vi "test_read-nmea-data2.vi"() -> ()   [LabVIEW 2019] (continued)
3,12,06,19,05,17,09,04,02,,,,,1.18,0.64,0.99,1*0A\n\t\n15:10:54.32\tF9P\t$GNGSA,A,3,85,71,84,,,,,,,,,,1.18,0.64,0.99,2*0F\n\t\n15:10:54.34\tF9P\t$GNGSA,A,3,36,19,11,04,09,12,,,,,,,1.18,0.64,0.99,3*0A\n\t\n15:10:54.37\tF9P\t$GNGSA,A,3,14,11,33,,,,,,,,,,1.18,0.64,0.99,4*0B\n\t\n15:10:54.39\tF9P\t$GPGSV,3,1,09,02,54,318,30,04,18,044,13,05,37,247,22,06,64,047,29,1*66\n\t\n15:10:54.41\tF9P\t$GPGSV,3,2,09,09,45,074,18,12,24,277,23,17,33,153,26,19,53,157,24,1*66\n\t\n15:10:54.43\tF9P\t$GPGSV,3,3,09,25,12,307,17,1*5B\n\t\n15:10:54.45\tF9P\t$GPGSV,3,1,09,02,54,318,,04,18,044,,05,37,247,,06,64,047,17,6*6D\n\t\n15:10:54.47\tF9P\t$GPGSV,3,2,09,09,45,074,,12,24,277,,17,33,153,15,19,53,157,,6*6F\n\t\n15:10:54.49\tF9P\t$GPGSV,3,3,09,25,12,307,,6*5A\n\t\n15:10:54.51\tF9P\t$GLGSV,2,1,08,69,12,031,,70,72,041,,71,51,205,16,72,03,209,,1*75\n\t\n15:10:54.53\tF9P\t$GLGSV,2,2,08,77,01,326,,84,20,122,11,85,70,065,23,86,36,330,,1*7A\n\t\n15:10:54.55\tF9P\t$GLGSV,2,1,08,69,12,031,,70,72,041,,71,51,205,23,72,03,209,,3*71\n\t\n15:10:54.57\tF9P\t$GLGSV,2,2,08,77,01,326,,84,20,122,15,85,70,065,21,86,36,330,,3*7E\n\t\n15:10:54.59\tF9P\t$GAGSV,2,1,08,02,09,298,11,04,66,119,25,09,31,193,21,11,71,357,20,7*7C\n\t\n15:10:54.61\tF9P\t$GAGSV,2,2,08,12,40,102,20,19,27,045,14,25,09,249,,36,25,308,10,7*7D\n\t\n15:10:54.63\tF9P\t$GAGSV,2,1,08,02,09,298,,04,66,119,24,09,31,193,,11,71,357,,2*79\n\t\n15:10:54.65\tF9P\t$GAGSV,2,2,08,12,40,102,29,19,27,045,,25,09,249,,36,25,308,,2*75\n\t\n15:10:54.67\tF9P\t$GBGSV,1,1,03,11,50,131,22,14,87,138,22,33,60,219,23,1*4E\n\t\n15:10:54.69\tF9P\t$GBGSV,1,1,03,11,50,131,35,14,87,138,15,33,60,219,,3*4F\n\t\n15:10:54.71\tF9P\t$GNGLL,3723.55311,N,12656.88974,E,061056.00,A,A*79\n\t\n15:10:54.73\tF9P\t\t\n15:10:54.75\tF9P\t\t\n15:10:54.77\tF9P\t\t\n15:10:54.79\tF9P\t\t\n15:10:54.81\tF9P\t\t\n15:10:54.83\tF9P\t\t\n15:10:54.85\tF9P\t\t\n15:10:54.87\tF9P\t\t\n15:10:54.89\tF9P\t\t\n15:10:54.91\tF9P\t\t\n15:10:54.93\tF9P\t\t\n15:10:54.95\tF9P\t\t\n15:10:54.97\tF9P\t\t\n15:10:54.99\tF9P\t\t\n15:10:55.01\tF9P\t\t\n15:10:55.03\tF9P\t\t\n15:10:55.05\tF9P\t\t\n15:10:55.07\tF9P\t\t\n15:10:55.09\tF9P\t\t\n15:10:55.11\tF9P\t\t\n15:10:55.13\tF9P\t\t\n15:10:55.15\tF9P\t\t\n15:10:55.17\tF9P\t\t\n15:10:55.19\tF9P\t\t\n15:10:55.21\tF9P\t\t\n15:10:55.23\tF9P\t\t\n15:10:55.25\tF9P\t$GNRMC,061057.00,A,3723.55267,N,12656.89064,E,2.717,135.11,250720,,,A,V*0A\n\t\n15:10:55.27\tF9P\t$GNVTG,135.11,T,,M,2.717,N,5.032,K,A*23\n\t\n15:10:55.29\tF9P\t$GNGGA,061057.00,3723.55267,N,12656.89064,E,1,12,0.64,66.5,M,18.5,M,,*7C\n\t\n15:10:55.31\tF9P\t$GNGSA,A,3,12,06,19,05,17,09,04,02,,,,,1.18,0.64,0.99,1*0A\n\t\n15:10:55.33\tF9P\t$GNGSA,A,3,85,71,84,,,,,,,,,,1.18,0.64,0.99,2*0F\n\t\n15:10:55.35\tF9P\t$GNGSA,A,3,36,19,11,04,09,12,,,,,,,1.18,0.64,0.99,3*0A\n\t\n15:10:55.37\tF9P\t$GNGSA,A,3,14,11,33,,,,,,,,,,1.18,0.64,0.99,4*0B\n\t\n15:10:55.39\tF9P\t$GPGSV,3,1,09,02,54,318,35,04,18,044,13,05,37,247,21,06,64,047,29,1*60\n\t\n15:10:55.41\tF9P\t$GPGSV,3,2,09,09,45,074,19,12,24,277,23,17,33,153,26,19,53,157,23,1*60\n\t\n15:10:55.43\tF9P\t$GPGSV,3,3,09,25,12,307,18,1*54\n\t\n15:10:55.45\tF9P\t$GPGSV,3,1,09,02,54,318,,04,18,044,,05,37,247,,06,64,047,17,6*6D\n\t\n15:10:55.47\tF9P\t$GPGSV,3,2,09,09,45,074,,12,24,277,,17,33,153,16,19,53,157,,6*6C\n\t\n15:10:55.49\tF9P\t$GPGSV,3,3,09,25,12,307,,6*5A\n\t\n15:10:55.51\tF9P\t$GLGSV,2,1,08,69,12,031,,70,72,041,,71,51,205,16,72,03,209,,1*75\n\t\n15:10:55.53\tF9P\t$GLGSV,2,2,08,77,01,326,,84,20,122,10,85,70,065,22,86,36,330,,1*7A\n\t\n15:10:55.55\tF9P\t$GLGSV,2,1,08,69,12,031,,70,72,041,,71,51,205,23,72,03,209,,3*71\n\t\n15:10:55.57\tF9P\t$GLGSV,2,2,08,77,01,326,,84,20,122,17,85,70,065,22,86,36,330,,3*7F\n\t\n15:10:55.59\tF9P\t$GAGSV,2,1,08,02,09,298,09,04,66,119,31,09,31,193,21,11,71,357,21,7*71\n\t\n15:10:55.61\tF9P\t$GAGSV,2,2,08,12,40,102,20,19,27,045,10,25,09,249,,36,25,308,10,7*79\n\t\n15:10:55.63\tF9P\t$GAGSV,2,1,08,02,09,298,,04,66,119,30,09,31,193,,11,71,357,,2*7C\n\t\n15:10:55.65\tF9P\t$GAGSV,2,2,08,12,40,102,26,19,27,045,,25,09,249,,36,25,308,,2*7A\n\t\n15:10:55.67\tF9P\t$GBGSV,1,1,03,11,50,131,24,14,87,138,21,33,60,219,23,1*4B\n\t\n15:10:55.69\tF9P\t$GBGSV,1,1,03,11,50,131,33,14,87,138,18,33,60,219,,3*44\n\t\n15:10:55.71\tF9P\t$GNGLL,3723.55267,N,12656.89064,E,061057.00,A,A*71\n\t\n15:10:55.73\tF9P\t\t\n15:10:55.75\tF9P\t\t\n15:10:55.77\tF9P\t\t\n15:10:55.79\tF9P\t\t\n15:10:55.81\tF9P\t\t\n15:10:55.83\tF9P\t\t\n15:10:55.85\tF9P\t\t\n15:10:55.87\tF9P\t\t\n15:10:55.89\tF9P\t\t\n15:10:55.91\tF9P\t\t\n15:10:55.93\tF9P\t\t\n15:10:55.95\tF9P\t\t\n15:10:55.97\tF9P\t\t\n15:10:55.99\tF9P\t\t\n15:10:56.01\tF9P\t\t\n15:10:56.03\tF9P\t\t\n15:10:56.05\tF9P\t\t\n15:10:56.07\tF9P\t\t\n15:10:56.09\tF9P\t\t\n15:10:56.11\tF9P\t\t\n15:10:56.13\tF9P\t\t\n15:10:56.15\tF9P\t\t\n15:10:56.17\tF9P\t\t\n15:10:56.19\tF9P\t\t\n15:10:56.21\tF9P\t\t\n15:10:56.23\tF9P\t\t\n15:10:56.25\tF9P\t$GNRMC,061058.00,A,3723.55188,N,12656.89111,E,3.072,148.78,250720,,,A,V*04\n\t\n15:10:56.27\tF9P\t$GNVTG,148.78,T,,M,3.072,N,5.690,K,A*2D\n\t\n15:10:56.29\tF9P\t$GNGGA,061058.00,3723.55188,N,12656.89111,E,1,12,0.76,66.2,M,18.5,M,,*76\n\t\n15:10:56.31\tF9P\t$GNGSA,A,3,12,06,19,05,17,09,04,02,,,,,1.40,0.76,1.18,1*0C\n\t\n15:10:56.33\tF9P\t$GNGSA,A,3,85,71,84,,,,,,,,,,1.40,0.76,1.18,2*09\n\t\n15:10:56.35\tF9P\t$GNGSA,A,3,36,19,11,04,09,12,,,,,,,1.40,0.76,1.18,3*0C\n\t\n15:10:56.37\tF9P\t$GNGSA,A,3,14,11,33,,,,,,,,,,1.40,0.76,1.18,4*0D\n\t\n15:10:56.39\tF9P\t$GPGSV,3,1,09,02,54,318,34,04,18,044,10,05,37,247,22,06,64,047,28,1*60\n\t\n15:10:56.41\tF9P\t$GPGSV,3,2,09,09,45,074,19,12,24,277,23,17,33,153,25,19,53,157,22,1*62\n\t\n15:10:56.43\tF9P\t$GPGSV,3,3,09,25,12,307,17,1*5B\n\t\n15:10:56.45\tF9P\t$GPGSV,3,1,09,02,54,318,,04,18,044,,05,37,247,,06,64,047,16,6*6C\n\t\n15:10:56.47\tF9P\t$GPGSV,3,2,09,09,45,074,,12,24,277,,17,33,153,18,19,53,157,,6*62\n\t\n15:10:56.49\tF9P\t$GPGSV,3,3,09,25,12,307,,6*5A\n\t\n15:10:56.51\tF9P\t$GLGSV,2,1,08,69,12,031,,70,72,041,,71,51,205,19,72,03,209,,1*7A\n\t\n15:10:56.53\tF9P\t$GLGSV,2,2,08,77,01,326,,84,20,122,09,85,70,065,22,86,36,330,,1*72\n\t\n15:10:56.55\tF9P\t$GLGSV,2,1,08,69,12,031,,70,72,041,,71,51,205,21,72,03,209,,3*73\n\t\n15:10:56.57\tF9P\t$GLGSV,2,2,08,77,01,326,,84,20,122,18,85,70,065,20,86,36,330,,3*72\n\t\n15:10:56.59\tF9P\t$GAGSV,2,1,08,02,09,298,11,04,66,119,25,09,31,193,20,11,71,357,22,7*7F\n\t\n15:10:56.61\tF9P\t$GAGSV,2,2,08,12,40,102,19,19,27,045,13,25,09,249,,36,25,308,14,7*74\n\t\n15:10:56.63\tF9P\t$GAGSV,2,1,08,02,09,298,,04,66,119,27,09,31,193,,11,71,357,,2*7A\n\t\n15:10:56.65\tF9P\t$GAGSV,2,2,08,12,40,102,26,19,27,045,,25,09,249,,36,25,308,,2*7A\n\t\n15:10:56.67\tF9P\t$GBGSV,1,1,03,11,50,131,24,14,87,138,21,33,60,219,21,1*49\n\t\n15:10:56.69\tF9P\t$GBGSV,1,1,03,11,50,131,33,14,87,138,21,33,60,219,,3*4E\n\t\n15:10:56.71\tF9P\t$GNGLL,3723.55188,N,12656.89111,E,061058.00,A,A*7F\n\t\n15:10:56.73\tF9P\t\t\n15:10:56.75\tF9P\t\t\n15:10:56.77\tF9P\t\t\n15:10:56.79\tF9P\t\t\n15:10:56.81\tF9P\t\t\n15:10:56.83\tF9P\t\t\n15:10:56.85\tF9P\t\t\n15:10:56.87\tF9P\t\t\n15:10:56.89\tF9P\t\t\n15:10:56.91\tF9P\t\t\n15:10:56.93\tF9P\t\t\n15:10:56.95\tF9P\t\t\n15:10:56.97\tF9P\t\t\n15:10:56.99\tF9P\t\t\n15:10:57.01\tF9P\t\t\n15:10:57.03\tF9P\t\t\n15:10:57.05\tF9P\t\t\n15:10:57.07\tF9P\t\t\n15:10:57.09\tF9P\t\t\n15:10:57.11\tF9P\t\t\n15:10:57.13\tF9P\t\t\n15:10:57.15\tF9P\t\t\n15:10:57.17\tF9P\t\t\n15:10:57.19\tF9P\t\t\n15:10:57.21\tF9P\t\t\n15:10:57.23\tF9P\t\t\n15:10:57.25\tF9P\t$GNRMC,061059.00,A,3723.55133,N,12656.89170,E,2.833,139.86,250720,,,A,V*09\n\t\n15:10:57.27\tF9P\t$GNVTG,139.86,T,,M,2.833,N,5.247,K,A*28\n\t\n15:10:57.29\tF9P\t$GNGGA,061059.00,3723.55133,N,12656.89170,E,1,12,0.67,66.6,M,18.5,M,,*74\n\t\n15:10:57.31\tF9P\t$GNGSA,A,3,12,06,19,05,17,09,04,02,,,,,1.23,0.67,1.03,1*03\n\t\n15:10:57.33\tF9P\t$GNGSA,A,3,85,71,84,,,,,,,,,,1.23,0.67,1.03,2*06\n\t\n15:10:57.35\tF9P\t$GNGSA,A,3,36,11,04,09,12,,,,,,,,1.23,0.67,1.03,3*0B\n\t\n15:10:57.37\tF9P\t$GNGSA,A,3,14,11,33,,,,,,,,,,1.23,0.67,1.03,4*02\n\t\n15:10:57.39\tF9P\t$GPGSV,3,1,09,02,54,318,36,04,18,044,11,05,37,247,22,06,64,047,29,1*62\n\t\n15:10:57.41\tF9P\t$GPGSV,3,2,09,09,45,074,19,12,24,277,22,17,33,153,26,19,53,157,22,1*60\n\t\n15:10:57.43\tF9P\t$GPGSV,3,3,09,25,12,307,16,1*5A\n\t\n15:10:57.45\tF9P\t$GPGSV,3,1,09,02,54,318,,04,18,044,,05,37,247,,06,64,047,15,6*6F\n\t\n15:10:57.47\tF9P\t$GPGSV,3,2,09,09,45,074,,12,24,277,,17,33,153,18,19,53,157,,6*62\n\t\n15:10:57.49\tF9P\t$GPGSV,3,3,09,25,12,307,,6*5A\n\t\n15:10:57.51\tF9P\t$GLGSV,2,1,08,69,12,031,,70,72,041,,71,51,205,19,72,03,209,,1*7A\n\t\n15:10:57.53\tF9P\t$GLGSV,2,2,08,77,01,326,,84,20,122,10,85,70,065,22,86,36,330,,1*7A\n\t\n15:10:57.55\tF9P\t$GLGSV,2,1,08,69,12,031,,70,72,041,,71,51,205,22,72,03,209,,3*70\n\t\n15:10:57.57\tF9P\t$GLGSV,2,2,08,77,01,326,,84,20,122,18,85,70,065,21,86,36,330,,3*73\n\t\n15:10:57.59\tF9P\t$GAGSV,2,1,08,02,08,297,07,04,66,119,30,09,31,193,19,11,71,357,22,7*78\n\t\n15:10:57.61\tF9P\t$GAGSV,2,2,08,12,40,102,18,19,27,045,07,25,09,249,,36,25,308,11,7*75\n\t\n15:10:57.63\tF9P\t$GAGSV,2,1,08,02,08,297,,04,66,119,26,09,31,193,,11,71,357,,2*75\n\t\n15:10:57.65\tF9P\t$GAGSV,2,2,08,12,40,102,25,19,27,045,,25,09,249,,36,25,308,,2*79\n\t\n15:10:57.67\tF9P\t$GBGSV,1,1,03,11,50,131,23,14,87,138,20,33,60,219,21,1*4F\n\t\n15:10:57.69\tF9P\t$GBGSV,1,1,03,11,50,131,29,14,87,138,20,33,60,219,,3*44\n\t\n15:10:57.71\tF9P\t$GNGLL,3723.55133,N,12656.89170,E,061059.00,A,A*79\n\t\n15:10:57.73\tF9P\t\t\n15:10:57.75\tF9P\t\t\n15:10:57.77\tF9P\t\t\n15:10:57.79\tF9P\t\t\n15:10:57.81\tF9P\t\t\n15:10:57.83\tF9P\t\t\n15:10:57.85\tF9P\t\t\n15:10:57.87\tF9P\t\t\n15:10:57.89\tF9P\t\t\n15:10:57.91\tF9P\t\t\n15:10:57.93\tF9P\t\t\n15:10:57.95\tF9P\t\t\n15:10:57.97\tF9P\t\t\n15:10:57.99\tF9P\t\t\n15:10:58.01\tF9P\t\t\n15:10:58.03\tF9P\t\t\n15:10:58.05\tF9P\t\t\n15:10:58.07\tF9P\t\t\n15:10:58.09\tF9P\t\t\n15:10:58.11\tF9P\t\t\n15:10:58.13\tF9P\t\t\n15:10:58.15\tF9P\t\t\n15:10:58.17\tF9P\t\t\n15:10:58.19\tF9P\t\t\n15:10:58.21\tF9P\t\t\n15:10:58.23\tF9P\t\t\n15:10:58.25\tF9P\t$GNRMC,061100.00,A,3723.55070,N,12656.89242,E,2.504,,250720,,,A,V*12\n\t\n15:10:58.27\tF9P\t$GNVTG,,T,,M,2.504,N,4.638,K,A*37\n\t\n15:10:58.29\tF9P\t$GNGGA,061100.00,3723.55070,N,12656.89242,E,1,12,0.68,66.4,M,18.5,M,,*70\n\t\n15:10:58.31\tF9P\t$GNGSA,A,3,12,06,19,05,17,09,02,,,,,,1.28,0.68,1.08,1*08\n\t\n15:10:58.33\tF9P\t$GNGSA,A,3,85,71,84,,,,,,,,,,1.28,0.68,1.08,2*09\n\t\n15:10:58.35\tF9P\t$GNGSA,A,3,36,19,11,04,09,12,,,,,,,1.28,0.68,1.08,3*0C\n\t\n15:10:58.37\tF9P\t$GNGSA,A,3,14,11,33,,,,,,,,,,1.28,0.68,1.08,4*0D\n\t\n15:10:58.39\tF9P\t$GPGSV,3,1,09,02,54,318,31,04,18,044,,05,37,247,22,06,64,047,28,1*64\n\t\n15:10:58.41\tF9P\t$GPGSV,3,2,09,09,45,074,18,12,24,277,22,17,33,153,26,19,53,157,22,1*61\n\t\n15:10:58.43\tF9P\t$GPGSV,3,3,09,25,12,307,15,1*59\n\t\n15:10:58.45\tF9P\t$GPGSV,3,1,09,02,54,318,,04,18,044,,05,37,247,,06,64,047,16,6*6C\n\t\n15:10:58.47\tF9P\t$GPGSV,3,2,09,09,45,074,,12,24,277,,17,33,153,17,19,53,157,,6*6D\n\t\n15:10:58.49\tF9P\t$GPGSV,3,3,09,25,12,307,,6*5A\n\t\n15:10:58.51\tF9P\t$GLGSV,2,1,08,69,12,031,,70,72,041,,71,51,205,18,72,03,209,,1*7B\n\t\n15:10:58.53\tF9P\t$GLGSV,2,2,08,77,01,326,,84,20,122,09,85,70,065,21,86,36,330,,1*71\n\t\n15:10:58.55\tF9P\t$GLGSV,2,1,08,69,12,031,,70,72,041,,71,51,205,21,72,03,209,,3*73\n\t\n15:10:58.57\tF9P\t$GLGSV,2,2,08,77,01,326,,84,20,122,17,85,70,065,20,86,36,330,,3*7D\n\t\n15:10:58.59\tF9P\t$GAGSV,2,1,08,02,08,297,07,04,66,119,22,09,31,193,18,11,71,357,21,7*79\n\t\n15:10:58.61\tF9P\t$GAGSV,2,2,08,12,40,102,20,19,27,045,07,25,09,249,,36,25,308,11,7*7E\n\t\n15:10:58.63\tF9P\t$GAGSV,2,1,08,02,08,297,,04,66,119,27,09,31,193,,11,71,357,,2*74\n\t\n15:10:58.65\tF9P\t$GAGSV,2,2,08,12,40,102,25,19,27,045,,25,09,249,,36,25,308,,2*79\n\t\n15:10:58.67\tF9P\t$GBGSV,1,1,03,11,50,131,22,14,87,138,20,33,60,219,22,1*4D\n\t\n15:10:58.69\tF9P\t$GBGSV,1,1,03,11,50,131,28,14,87,138,22,33,60,219,,3*47\n\t\n15:10:58.71\tF9P\t$GNGLL,3723.55070,N,12656.89242,E,061100.00,A,A*70\n\t\n15:10:58.73\tF9P\t\t\n15:10:58.75\tF9P\t\t\n15:10:58.77\tF9P\t\t\n15:10:58.79\tF9P\t\t\n15:10:58.81\tF9P\t\t\n15:10:58.83\tF9P\t\t\n15:10:58.85\tF9P\t\t\n15:10:58.87\tF9P\t\t\n15:10:58.89\tF9P\t\t\n15:10:58.91\tF9P\t\t\n15:10:58.93\tF9P\t\t\n15:10:58.95\tF9P\t\t\n15:10:58.97\tF9P\t\t\n15:10:58.99\tF9P\t\t\n15:10:59.01\tF9P\t\t\n15:10:59.03\tF9P\t\t\n15:10:59.05\tF9P\t\t\n15:10:59.07\tF9P\t\t\n15:10:59.09\tF9P\t\t\n15:10:59.11\tF9P\t\t\n15:10:59.13\tF9P\t\t\n15:10:59.15\tF9P\t\t\n15:10:59.17\tF9P\t\t\n15:10:59.19\tF9P\t\t\n15:10:59.21\tF9P\t\t\n15:10:59.23\tF9P\t\t\n15:10:59.25\tF9P\t$GNRMC,061101.00,A,3723.55024,N,12656.89321,E,2.638,134.57,250720,,,A,V*00\n\t\n15:10:59.27\tF9P\t$GNVTG,134.57,T,,M,2.638,N,4.886,K,A*2A\n\t\n15:10:59.29\tF9P\t$GNGGA,061101.00,3723.55024,N,12656.89321,E,1,12,0.76,64.9,M,18.5,M,,*74\n\t\n15:10:59.31\tF9P\t$GNGSA,A,3,12,06,19,05,17,09,02,,,,,,1.40,0.76,1.18,1*08\n\t\n15:10:59.33\tF9P\t$GNGSA,A,3,85,71,84,,,,,,,,,,1.40,0.76,1.18,2*09\n\t\n15:10:59.35\tF9P\t$GNGSA,A,3,36,19,11,04,09,12,,,,,,,1.40,0.76,1.18,3*0C\n\t\n15:10:59.37\tF9P\t$GNGSA,A,3,14,11,33,,,,,,,,,,1.40,0.76,1.18,4*0D\n\t\n15:10:59.39\tF9P\t$GPGSV,3,1,09,02,54,318,34,04,18,044,,05,37,247,22,06,64,047,27,1*6E\n\t\n15:10:59.41\tF9P\t$GPGSV,3,2,09,09,45,074,18,12,24,277,22,17,33,153,27,19,53,157,22,1*60\n\t\n15:10:59.43\tF9P\t$GPGSV,3,3,09,25,12,307,15,1*59\n\t\n15:10:59.45\tF9P\t$GPGSV,3,1,09,02,54,318,,04,18,044,,05,37,247,,06,64,047,16,6*6C\n\t\n15:10:59.47\tF9P\t$GPGSV,3,2,09,09,45,074,,12,24,277,,17,33,153,16,19,53,157,,6*6C\n\t\n15:10:59.49\tF9P\t$GPGSV,3,3,09,25,12,307,,6*5A\n\t\n15:10:59.51\tF9P\t$GLGSV,2,1,08,69,12,031,,70,72,041,,71,51,205,19,72,03,209,,1*7A\n\t\n15:10:59.53\tF9P\t$GLGSV,2,2,08,77,01,326,,84,20,122,10,85,70,065,21,86,36,330,,1*79\n\t\n15:10:59.55\tF9P\t$GLGSV,2,1,08,69,12,031,,70,72,041,,71,51,205,21,72,03,209,,3*73\n\t\n15:10:59.57\tF9P\t$GLGSV,2,2,08,77,01,326,,84,20,122,15,85,70,065,19,86,36,330,,3*75\n\t\n15:10:59.59\tF9P\t$GAGSV,2,1,08,02,08,297,09,04,66,118,27,09,31,193,17,11,71,357,20,7*7D\n\t\n15:10:59.61\tF9P\t$GAGSV,2,2,08,12,40,102,19,19,27,045,13,25,09,249,,36,25,308,11,7*71\n\t\n15:10:59.63\tF9P\t$GAGSV,2,1,08,02,08,297,,04,66,118,27,09,31,193,,11,71,357,,2*75\n\t\n15:10:59.65\tF9P\t$GAGSV,2,2,08,12,40,102,24,19,27,045,,25,09,249,,36,25,308,,2*78\n\t\n15:10:59.67\tF9P\t$GBGSV,1,1,03,11,50,131,21,14,87,138,21,33,60,219,22,1*4F\n\t\n15:10:59.69\tF9P\t$GBGSV,1,1,03,11,50,131,,14,87,138,22,33,60,219,,3*4D\n\t\n15:10:59.71\tF9P\t$GNGLL,3723.55024,N,12656.89321,E,061101.00,A,A*74\n\t\n15:10:59.73\tF9P\t\t\n15:10:59.75\tF9P\t\t\n15:10:59.77\tF9P\t\t\n15:10:59.79\tF9P\t\t\n15:10:59.81\tF9P\t\t\n15:10:59.83\tF9P\t\t\n15:10:59.85\tF9P\t\t\n15:10:59.87\tF9P\t\t\n15:10:59.89\tF9P\t\t\n15:10:59.91\tF9P\t\t\n15:10:59.93\tF9P\t\t\n15:10:59.95\tF9P\t\t\n15:10:59.97\tF9P\t\t\n15:10:59.99\tF9P\t\t\n15:11:00.01\tF9P\t\t\n15:11:00.03\tF9P\t\t\n15:11:00.05\tF9P\t\t\n15:11:00.07\tF9P\t\t\n15:11:00.09\tF9P\t\t\n15:11:00.11\tF9P\t\t\n15:11:00.13\tF9P\t\t\n15:11:00.15\tF9P\t\t\n15:11:00.17\tF9P\t\t\n15:11:00.19\tF9P\t\t\n15:11:00.21\tF9P\t\t\n15:11:00.23\tF9P\t\t\n15:11:00.25\tF9P\t$GNRMC,061102.00,A,3723.54956,N,12656.89368,E,2.597,143.40,250720,,,A,V*03\n\t\n15:11:00.27\tF9P\t$GNVTG,143.40,T,,M,2.597,N,4.810,K,A*25\n\t\n15:11:00.29\tF9P\t$GNGGA,061102.00,3723.54956,N,12656.89368,E,1,12,0.68,64.8,M,18.5,M,,*79\n\t\n15:11:00.31\tF9P\t$GNGSA,A,3,12,06,19,05,17,09,02,,,,,,1.28,0.68,1.08,1*08\n\t\n15:11:00.33\tF9P\t$GNGSA,A,3,85,71,84,,,,,,,,,,1.28,0.68,1.08,2*09\n\t\n15:11:00.35\tF9P\t$GNGSA,A,3,36,19,11,04,09,12,,,,,,,1.28,0.68,1.08,3*0C\n\t\n15:11:00.37\tF9P\t$GNGSA,A,3,14,11,33,,,,,,,,,,1.28,0.68,1.08,4*0D\n\t\n15:11:00.39\tF9P\t$GPGSV,3,1,09,02,54,318,35,04,18,044,,05,37,247,22,06,64,047,27,1*6F\n\t\n15:11:00.41\tF9P\t$GPGSV,3,2,09,09,45,074,19,12,24,277,23,17,33,153,26,19,53,157,22,1*61\n\t\n15:11:00.43\tF9P\t$GPGSV,3,3,09,25,12,307,16,1*5A\n\t\n15:11:00.45\tF9P\t$GPGSV,3,1,09,02,54,318,,04,18,044,,05,37,247,,06,64,047,14,6*6E\n\t\n15:11:00.47\tF9P\t$GPGSV,3,2,09,09,45,074,,12,24,277,,17,33,153,15,19,53,157,,6*6F\n\t\n15:11:00.49\tF9P\t$GPGSV,3,3,09,25,12,307,,6*5A\n\t\n15:11:00.51\tF9P\t$GLGSV,2,1,08,69,12,031,,70,72,041,,71,51,205,18,72,03,209,,1*7B\n\t\n15:11:00.53\tF9P\t$GLGSV,2,2,08,77,01,326,,84,20,122,11,85,70,065,21,86,36,330,,1*78\n\t\n15:11:00.55\tF9P\t$GLGSV,2,1,08,69,12,031,,70,72,041,,71,51,205,20,72,03,209,,3*72\n\t\n15:11:00.57\tF9P\t$GLGSV,2,2,08,77,01,326,,84,20,122,14,85,70,065,20,86,36,330,,3*7E\n\t\n15:11:00.59\tF9P\t$GAGSV,2,1,08,02,08,297,07,04,66,118,25,09,31,193,16,11,71,357,19,7*7A\n\t\n15:11:00.61\tF9P\t$GAGSV,2,2,08,12,40,102,18,19,27,045,09,25,09,249,,36,25,308,14,7*7E\n\t\n15:11:00.63\tF9P\t$GAGSV,2,1,08,02,08,297,,04,66,118,26,09,31,193,,11,71,357,,2*74\n\t\n15:11:00.65\tF9P\t$GAGSV,2,2,08,12,40,102,29,19,27,045,,25,09,249,,36,25,308,,2*75\n\t\n15:11:00.67\tF9P\t$GBGSV,1,1,03,11,50,131,20,14,87,138,21,33,60,219,21,1*4D\n\t\n15:11:00.69\tF9P\t$GBGSV,1,1,03,11,50,131,28,14,87,138,22,33,60,219,,3*47\n\t\n15:11:00.71\tF9P\t$GNGLL,3723.54956,N,12656.89368,E,061102.00,A,A*77\n\t\n15:11:00.73\tF9P\t\t\n15:11:00.75\tF9P\t\t\n15:11:00.77\tF9P\t\t\n15:11:00.79\tF9P\t\t\n15:11:00.81\tF9P\t\t\n15:11:00.83\tF9P\t\t\n15:11:00.85\tF9P\t\t\n15:11:00.87\tF9P\t\t\n15:11:00.89\tF9P\t\t\n15:11:00.91\tF9P\t\t\n15:11:00.93\tF9P\t\t\n15:11:00.95\tF9P\t\t\n15:11:00.97\tF9P\t\t\n15:11:00.99\tF9P\t\t\n15:11:01.01\tF9P\t\t\n15:11:01.03\tF9P\t\t\n15:11:01.05\tF9P\t\t\n15:11:01.07\tF9P\t\t\n15:11:01.09\tF9P\t\t\n15:11:01.11\tF9P\t\t\n15:11:01.13\tF9P\t\t\n15:11:01.15\tF9P\t\t\n15:11:01.17\tF9P\t\t\n15:11:01.19\tF9P\t\t\n15:11:01.21\tF9P\t\t\n15:11:01.23\tF9P\t\t\n15:11:01.25\tF9P\t$GNRMC,061103.00,A,3723.54923,N,12656.89425,E,2.106,,250720,,,A,V*1E\n\t\n15:11:01.27\tF9P\t$GNVTG,,T,,M,2.106,N,3.901,K,A*33\n\t\n15:11:01.29\tF9P\t$GNGGA,061103.00,3723.54923,N,12656.89425,E,1,12,0.68,65.3,M,18.5,M,,*7E\n\t\n15:11:01.31\tF9P\t$GNGSA,A,3,12,06,19,05,17,09,02,,,,,,1.28,0.68,1.08,1*08\n\t\n15:11:01.33\tF9P\t$GNGSA,A,3,85,71,84,,,,,,,,,,1.28,0.68,1.08,2*09\n\t\n15:11:01.35\tF9P\t$GNGSA,A,3,36,19,11,04,09,12,,,,,,,1.28,0.68,1.08,3*0C\n\t\n15:11:01.37\tF9P\t$GNGSA,A,3,14,11,33,,,,,,,,,,1.28,0.68,1.08,4*0D\n\t\n15:11:01.39\tF9P\t$GPGSV,3,1,09,02,54,318,34,04,18,044,,05,37,247,21,06,64,047,32,1*69\n\t\n15:11:01.41\tF9P\t$GPGSV,3,2,09,09,45,074,18,12,24,277,22,17,33,153,24,19,53,157,21,1*60\n\t\n15:11:01.43\tF9P\t$GPGSV,3,3,09,25,12,307,,1*5D\n\t\n15:11:01.45\tF9P\t$GPGSV,3,1,09,02,54,318,,04,18,044,,05,37,247,,06,64,047,,6*6B\n\t\n15:11:01.47\tF9P\t$GPGSV,3,2,09,09,45,074,,12,24,277,,17,33,153,13,19,53,157,,6*69\n\t\n15:11:01.49\tF9P\t$GPGSV,3,3,09,25,12,307,,6*5A\n\t\n15:11:01.51\tF9P\t$GLGSV,2,1,08,69,12,031,,70,72,041,,71,51,205,16,72,03,209,,1*75\n\t\n15:11:01.53\tF9P\t$GLGSV,2,2,08,77,01,326,,84,20,122,08,85,70,065,22,86,36,330,,1*73\n\t\n15:11:01.55\tF9P\t$GLGSV,2,1,08,69,12,031,,70,72,041,,71,51,205,19,72,03,209,,3*78\n\t\n15:11:01.57\tF9P\t$GLGSV,2,2,08,77,01,326,,84,20,122,16,85,70,065,20,86,36,330,,3*7C\n\t\n15:11:01.59\tF9P\t$GAGSV,2,1,08,02,08,297,08,04,66,118,25,09,31,193,17,11,71,357,19,7*74\n\t\n15:11:01.61\tF9P\t$GAGSV,2,2,08,12,40,102,18,19,27,045,10,25,09,249,,36,25,308,18,7*7A\n\t\n15:11:01.63\tF9P\t$GAGSV,2,1,08,02,08,297,,04,66,118,25,09,31,193,,11,71,357,,2*77\n\t\n15:11:01.65\tF9P\t$GAGSV,2,2,08,12,40,102,27,19,27,045,,25,09,249,,36,25,308,,2*7B\n\t\n15:11:01.67\tF9P\t$GBGSV,1,1,03,11,50,131,19,14,87,138,22,33,60,219,21,1*44\n\t\n15:11:01.69\tF9P\t$GBGSV,1,1,03,11,50,131,32,14,87,138,20,33,60,219,,3*4E\n\t\n15:11:01.71\tF9P\t$GNGLL,3723.54923,N,12656.89425,E,061103.00,A,A*7A\n\t\n15:11:01.73\tF9P\t\t\n15:11:01.75\tF9P\t\t\n15:11:01.77\tF9P\t\t\n15:11:01.79\tF9P\t\t\n15:11:01.81\tF9P\t\t\n15:11:01.83\tF9P\t\t\n15:11:01.85\tF9P\t\t\n15:11:01.87\tF9P\t\t\n15:11:01.89\tF9P\t\t\n15:11:01.91\tF9P\t\t\n15:11:01.93\tF9P\t\t\n15:11:01.95\tF9P\t\t\n15:11:01.97\tF9P\t\t\n15:11:01.99\tF9P\t\t\n15:11:02.01\tF9P\t\t\n15:11:02.03\tF9P\t\t\n15:11:02.05\tF9P\t\t\n15:11:02.07\tF9P\t\t\n15:11:02.09\tF9P\t\t\n15:11:02.11\tF9P\t\t\n15:11:02.13\t
